vi "Bounds Separator.vi"(8 "error in (no error)":errorcluster, 10 "Boolean":bool, 11 "GObjct in":refnum<class "GObject.lvclass">) -> (0 "error out":errorcluster, 3 "GObjct out":refnum<class "GObject.lvclass">)   [LabVIEW 2015, in "GObject.lvclass"]
uses:
  GObject.lvclass
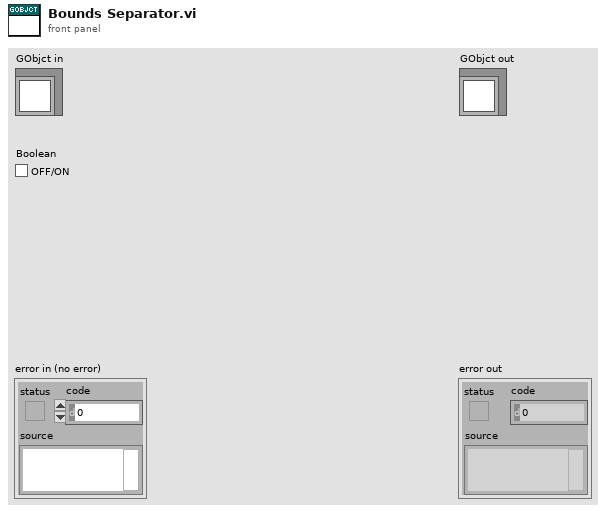
[diagram p1: front panel]
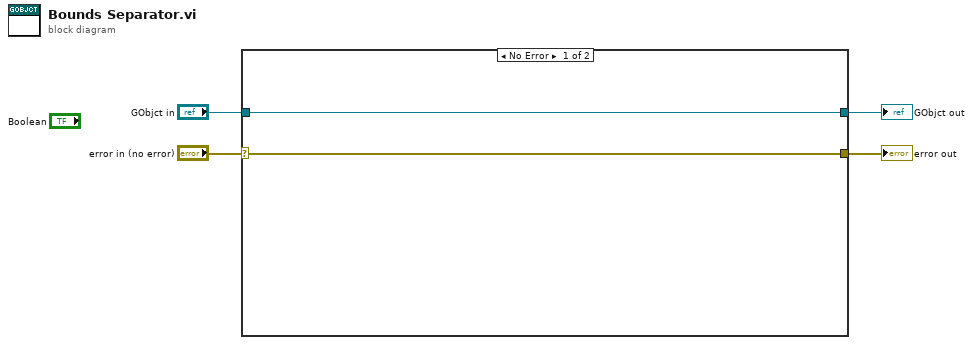
[diagram p0: block diagram]
diagram:
  n1 = case shown="No Error" "error in (no error)" {
    selector: "error in (no error)" -> [w5 w8]
    tunnel: [w5 w8] -> w3
    tunnel: [w6 w7] -> w1
    tunnel: "GObjct in" -> [w6 w7]
    frame No Error {
    }
    frame Error {
    }
  }
  "error out" <- w3
  "GObjct out" <- w1
